vi "Get Mass.vi"(8 "error in (no error)":errorcluster, 11 "Link in":refnum<class "Link.lvclass">) -> (0 "error out":errorcluster, 2 "Mass":dbl, 3 "Link out":refnum<class "Link.lvclass">)   [LabVIEW 2013, in "Link.lvclass"]
uses:
  Link.lvclass
  Link.lvclass/Link.ctl
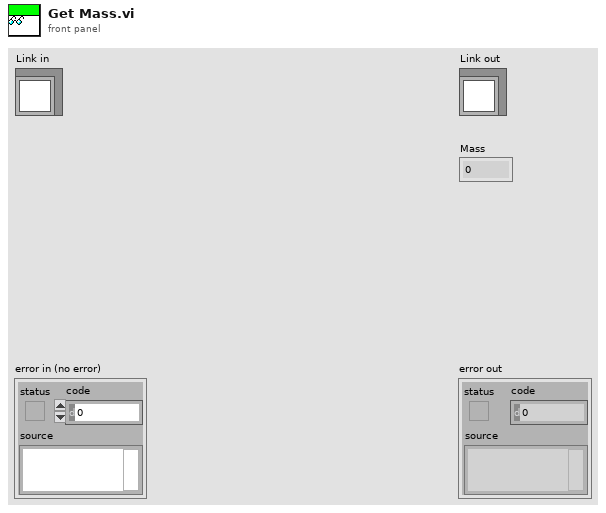
[diagram p1: front panel]
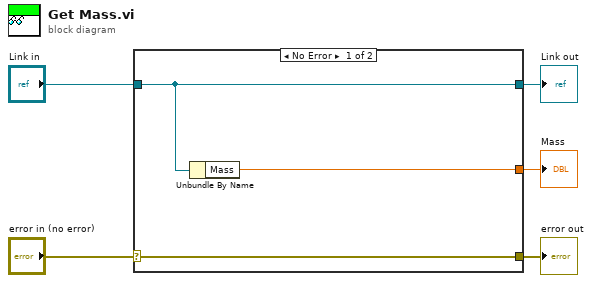
[diagram p0: block diagram]
diagram:
  n1 = case shown="No Error" "error in (no error)" {
    selector: "error in (no error)" -> [w8 w9]
    tunnel: [w8 w9] -> w4
    tunnel: [w7 w10] -> w2
    tunnel: "Link in" -> [w7 w10]
    tunnel: [w6 _] -> w1
    frame No Error {
      n2 = Unbundle By Name(w7) -> ("Mass"=w6:dbl)
    }
    frame Error {
    }
  }
  "error out" <- w4
  "Link out" <- w2
  "Mass" <- w1
